vi "Initialize.vi"(0 "Yokogawa WT2X0 in":refnum<class "Yokogawa WT2X0.lvclass">, 7 "Reset (T: Reset)":bool=TRUE, 9 "ID Query (T: Check)":bool, 11 "error in (no error)":errorcluster) -> (4 "Yokogawa WT2X0 out":refnum<class "Yokogawa WT2X0.lvclass">, 6 "VISA resource name":refnum<visa-resource-name>, 15 "error out":errorcluster)   [LabVIEW 2013, in "Universal Power Meter.lvlib" / "Yokogawa WT2X0.lvlib" / "Yokogawa WT2X0.lvclass"]
uses:
  Yokogawa WT2X0.lvclass
  Universal Power Meter class/Universal Power Meter.lvclass
  <instrlib>/Yokogawa WT200 Series/Yokogawa WT200 Series.lvlib
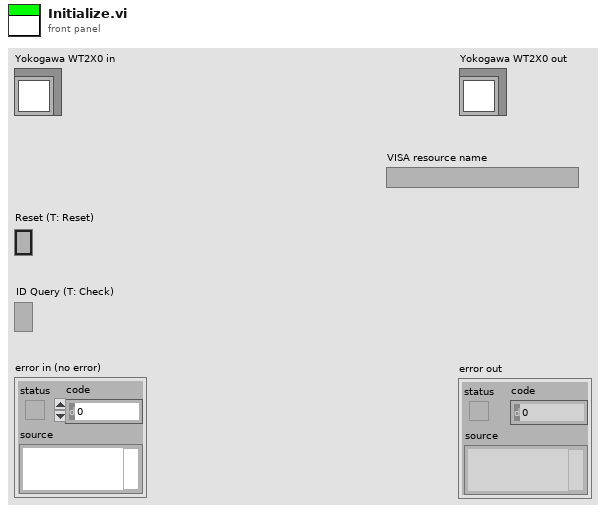
[diagram p1: front panel]
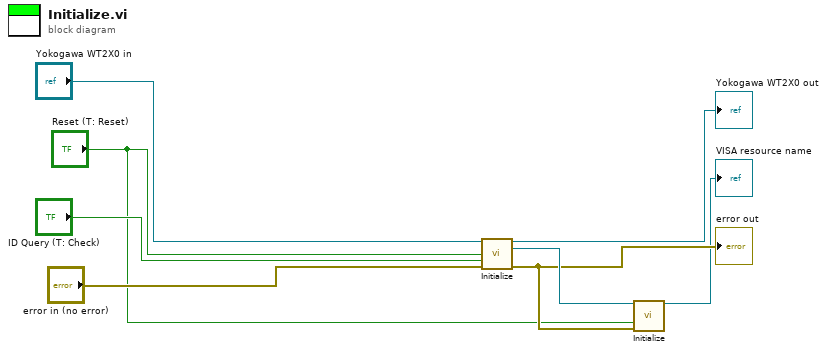
[diagram p0: block diagram]
diagram:
  n1 = call-parent <instrlib>:"Initialize.vi"("Universal Power Meter in"="Yokogawa WT2X0 in", "Reset (T: Reset)"="Reset (T: Reset)", "ID Query (T: Check)"="ID Query (T: Check)", "error in (no error)"="error in (no error)") -> ("Universal Power Meter out"=→"Yokogawa WT2X0 out":refnum<class "Yokogawa WT2X0.lvclass">, "VISA resource name"=w4:refnum<visa-resource-name>, "error out"=w3:errorcluster)  [unwired: 9 in]
  "error out" <- w3
  n2 = call <instrlib>:"Initialize.vi"("VISA resource name"=w4, "Reset (T: Reset)"="Reset (T: Reset)", "error in (no error)"=w3) -> ("VISA resource name out"=→"VISA resource name":refnum<visa-resource-name>)  [unwired: 11 in, 1 out]
